vi "mod_Rician Selective Fading (Jakes).vi"(0 "profile length (samples)":i32=1000, 1 "rician parameter K (dB)":dbl=1.0 format="%.2f", 2 "number of paths":i32=1, 5 "sampling frequency (Hz)":dbl=1.0 format="%.2f", 7 "doppler spread (Hz)":dbl=0.01 format="%.2p", 9 "seed in (0xFFFFFFFF)":i32=-1 format="%.0x", 11 "error in (no error)":errorcluster, 12 "fading variance":dbl=1.0 format="%.2f", 13 "reset? (T)":bool=TRUE) -> (4 "Rician Fading profile":cdb[][](array[numeric]), 10 "next seed":i32=-1 format="%.0x", 15 "error out":errorcluster)   [LabVIEW 2020, in "niDMT.lvlib"]
uses:
  <vilib>/addons/Modulation/niDMT.lvlib
  <vilib>/addons/Modulation/niAMT.lvlib
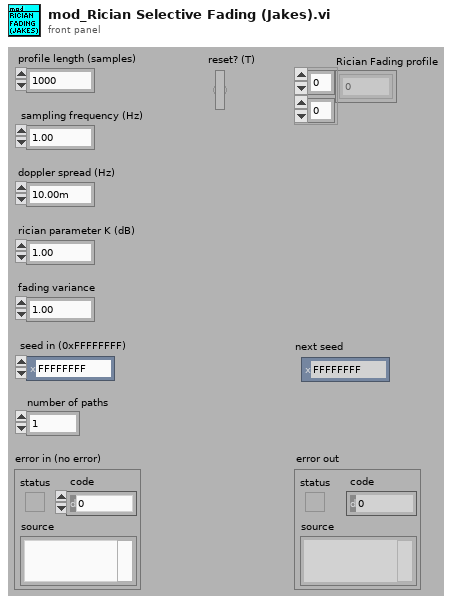
[diagram p1: front panel]
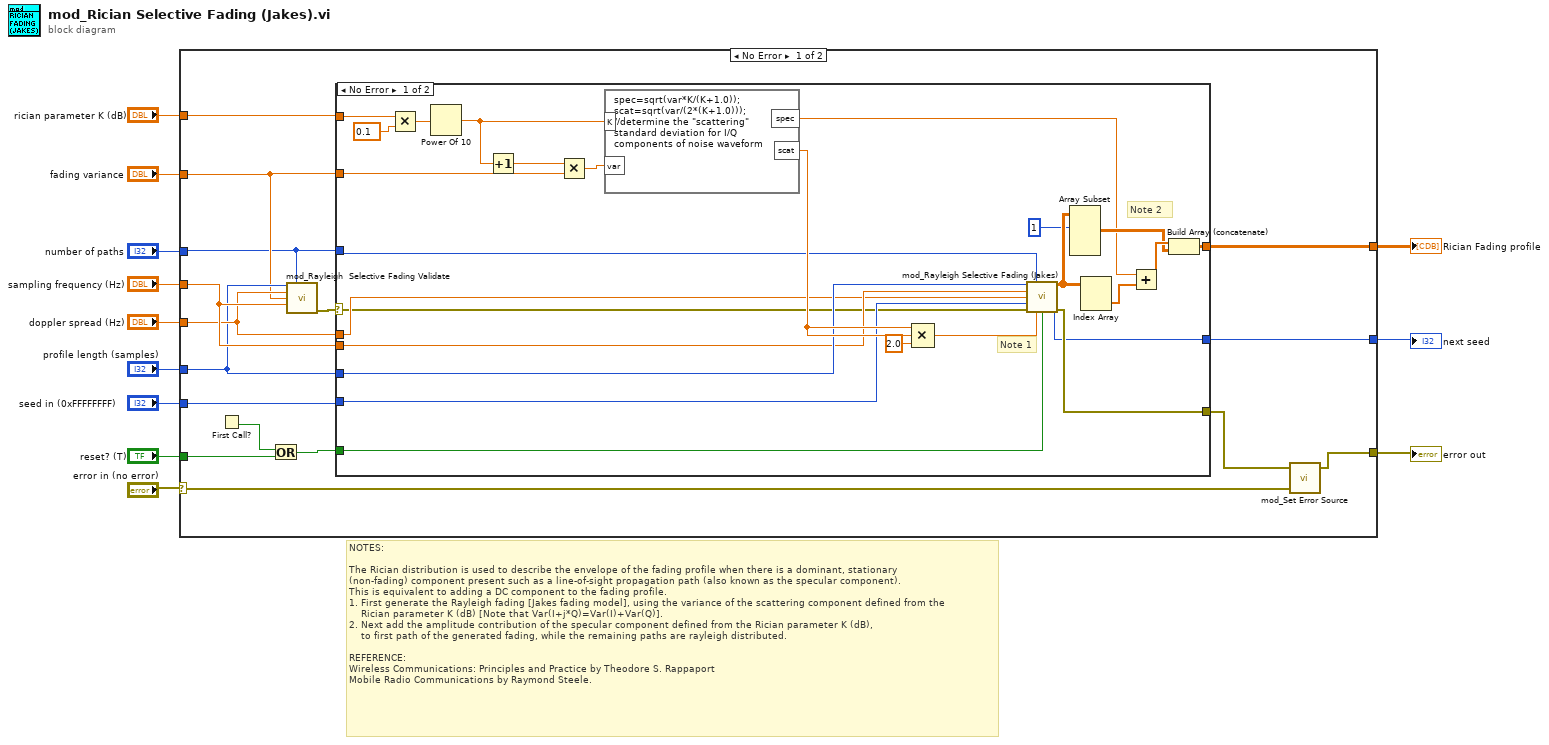
[diagram p0: block diagram]
diagram:
  # "NOTES:\n\nThe Rician distribution is used to describe the envelope of the fading profile when there is a dominant, stationary\n(non-fading) component present such as a line-of-sight propagation path (also known as the specular component).\nThis is equivalent to adding a DC component to the fading profile.\n1. First generate the Rayleigh fading [Jakes fading model], using the variance of the scattering component defined from the\n    Rician parameter K (dB) [Note that Var(I+j*Q)=Var(I)+Var(Q)].\n2. Next add the amplitude contribution of the specular component defined from the Rician parameter K (dB),\n    to first path of the generated fading, while the remaining paths are rayleigh distributed.\n\nREFERENCE:\nWireless Communications: Principles and Practice by Theodore S. Rappaport\nMobile Radio Communications by Raymond Steele."
  n1 = case shown="No Error" "error in (no error)" {
    selector: "error in (no error)" -> [w27 w56]
    tunnel: [w28 w56] -> w12
    tunnel: "rician parameter K (dB)" -> [w15 _]
    tunnel: "sampling frequency (Hz)" -> [w23 _]
    tunnel: "doppler spread (Hz)" -> [w22 _]
    tunnel: "profile length (samples)" -> [w21 _]
    tunnel: "seed in (0xFFFFFFFF)" -> [w20 _]
    tunnel: "reset? (T)" -> [w18 _]
    tunnel: "fading variance" -> [w17 _]
    tunnel: [w16 _] -> w3
    tunnel: "number of paths" -> [w13 _]
    tunnel: [w14 _] -> w1
    frame No Error {
      n2 = First Call?() -> (First Call?: T/F=w19:bool)
      n3 = Or(x=w19, y=w18) -> (x .or. y?=w24:bool)
      n4 = call <vilib>:"mod_Rayleigh  Selective Fading Validate.vi"("profile length (samples)"=w21, "paths"=w13, "doppler spread (Hz)"=w22, "fading variance"=w17, "sampling frequency"=w23) -> ("error out"=w25:errorcluster)  [unwired: 10 out]
      n5 = case shown="No Error" w25 {
        selector: w25 -> [w41 w55]
        tunnel: w22 -> [w43 _]
        tunnel: w21 -> [w45 _]
        tunnel: [w38 w55] -> w26
        tunnel: w23 -> [w44 _]
        tunnel: w15 -> [w52 _]
        tunnel: w24 -> [w39 _]
        tunnel: w20 -> [w42 _]
        tunnel: w17 -> [w47 _]
        tunnel: [w37 _] -> w16
        tunnel: w13 -> [w36 _]
        tunnel: [w30 _] -> w14
        frame No Error {
          # "Note 2"
          # "Note 1"
          n6 = Multiply(x=w52, y=0.1) -> (x*y=w54:dbl)
          n7 = Power Of 10(x=w54) -> (10^x=w49:dbl)
          n8 = Increment(x=w49) -> (x+1=w48:dbl)
          n9 = Multiply(x=w48, y=w47) -> (x*y=w46:dbl)
          n10 = formula code="spec=sqrt(var*K/(K+1.0));\nscat=sqrt(var/(2*(K+1.0)));\n//determine the \"scattering\" standard deviation for I/Q components of noise waveform"("K"=w49, "var"=w46) -> ("scat"=w51:dbl, "spec"=w29:dbl)
          n11 = Compound Arithmetic op=MULTIPLY(w51, w51, 2.0 ("value")) -> (w40:dbl)
          n12 = call <vilib>:"mod_Rayleigh Selective Fading (Jakes).vi"("profile length (samples)"=w45, "number of paths"=w36, "sampling frequency (Hz)"=w44, "doppler spread (Hz)"=w43, "seed in (0xFFFFFFFF)"=w42, "error in (no error)"=w41, "fading variance"=w40, "reset? (T)"=w39) -> ("fading profile"=w34:cdb[][], "next seed"=w37:i32, "error out"=w38:errorcluster)  [unwired: 5 out]
          n13 = Array Subset(array=w34, index (row)=1 ("index")) -> (w31:cdb[][])  [unwired: 3 in]
          n14 = Index Array(array=w34) -> (element=w35:cdb[])  [unwired: 2 in]
          n15 = Add(x=w29, y=w35) -> (x+y=w32:cdb[])
          n16 = Build Array (concatenate)(w32, w31) -> (w30:cdb[][])
        }
        frame Error {
        }
      }
      n17 = call <vilib>:"mod_Set Error Source.vi"("initial error in (no error)"=w27, "final error in (no error)"=w26) -> ("error out"=w28:errorcluster)  [unwired: 1 in, 2 out]
    }
    frame Error {
    }
  }
  "error out" <- w12
  "next seed" <- w3
  "Rician Fading profile" <- w1
